vi "FPGA port check.vi"() -> ()   [LabVIEW 2009]
uses:
  <vilib>/eio/EIONode/EIONode.xnode
  <vilib>/rvi/eio/nirviEIOImplementation/nirviEIOImplementation.xnode
  <vilib>/rvi/eio/common/nirviEmuTemplateMethod_noerrors.vi
  <vilib>/rvi/eio/common/nirviEmuClasses.ctl
panel:
  in  "stop":bool
  out "Port4/DIOCTL":bool
  out "Port3/DIOCTL":bool
  out "Port7/DIO9":bool
  out "Port7/DIO0":bool
  out "Port7/DIO1":bool
  out "Port7/DIO2":bool
  out "Port7/DIO3":bool
  out "Port4/DIO9":bool
  out "Port3/DIO9":bool
  out "Port3/DIO0":bool
  out "Port3/DIO1":bool
  out "Port3/DIO2":bool
  out "Port3/DIO3":bool
  out "Port3/DIO4":bool
  out "Port3/DIO5":bool
  out "Port3/DIO6":bool
  out "Port3/DIO7":bool
  out "Port3/DIO8":bool
  out "Port4/DIO0":bool
  out "Port4/DIO1":bool
  out "Port4/DIO2":bool
  out "Port4/DIO3":bool
  out "Port4/DIO4":bool
  out "Port4/DIO6":bool
  out "Port4/DIO8":bool
  out "Port4/DIO7":bool
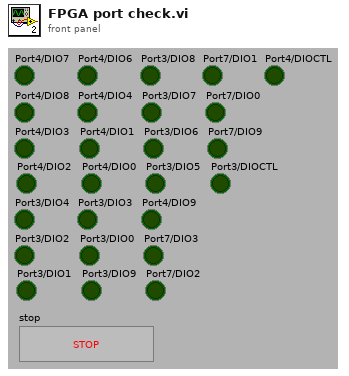
[diagram p1: front panel]
types:
  T1 = typedef "nirviEmuClasses.ctl" = enum16{"IO Read", "IO Write", "Method", "Property Read", "Property Write"}
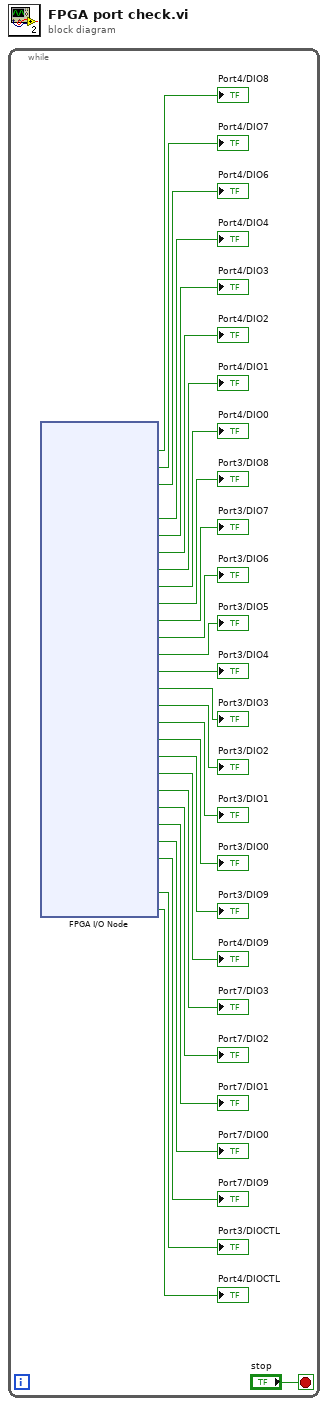
[diagram p0: block diagram]
diagram:
  n1 = while {
    stop <- "stop" stop-if-true
    n2 = xnode "FPGA I/O Node"() -> ("Port4/DIO8"=→"Port4/DIO8":bool, "Port4/DIO7"=→"Port4/DIO7":bool, "Port4/DIO6"=→"Port4/DIO6":bool, "Port4/DIO4"=→"Port4/DIO4":bool, "Port4/DIO3"=→"Port4/DIO3":bool, "Port4/DIO2"=→"Port4/DIO2":bool, "Port4/DIO1"=→"Port4/DIO1":bool, "Port4/DIO0"=→"Port4/DIO0":bool, "Port3/DIO8"=→"Port3/DIO8":bool, "Port3/DIO7"=→"Port3/DIO7":bool, "Port3/DIO6"=→"Port3/DIO6":bool, "Port3/DIO5"=→"Port3/DIO5":bool, "Port3/DIO4"=→"Port3/DIO4":bool, "Port3/DIO3"=→"Port3/DIO3":bool, "Port3/DIO2"=→"Port3/DIO2":bool, "Port3/DIO1"=→"Port3/DIO1":bool, "Port3/DIO0"=→"Port3/DIO0":bool, "Port3/DIO9"=→"Port3/DIO9":bool, "Port4/DIO9"=→"Port4/DIO9":bool, "Port7/DIO3"=→"Port7/DIO3":bool, "Port7/DIO2"=→"Port7/DIO2":bool, "Port7/DIO1"=→"Port7/DIO1":bool, "Port7/DIO0"=→"Port7/DIO0":bool, "Port7/DIO9"=→"Port7/DIO9":bool, "Port3/DIOCTL"=→"Port3/DIOCTL":bool, "Port4/DIOCTL"=→"Port4/DIOCTL":bool)  [unwired: 28 in, 30 out]
  }
